vi "Write Image Name.vi"(8 "error in (no error)":errorcluster, 10 "Image Name":string, 11 "CCD in":refnum<class "CCD.lvclass">) -> (0 "error out":errorcluster, 3 "CCD out":refnum<class "CCD.lvclass">)   [LabVIEW 2018, in "CCD.lvclass"]
uses:
  CCD.lvclass
  CCD.lvclass/CCD.ctl
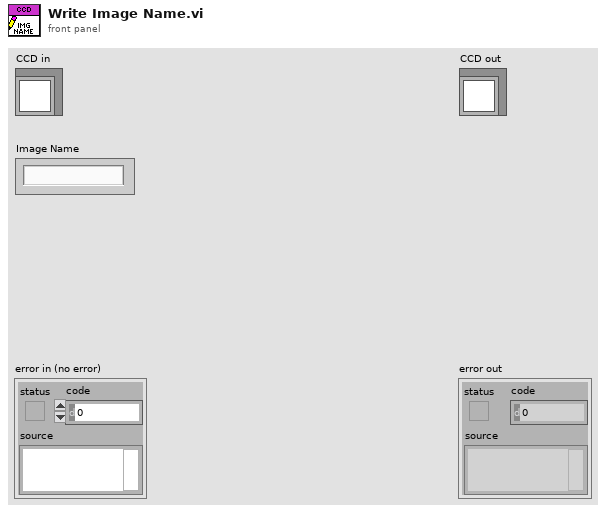
[diagram p1: front panel]
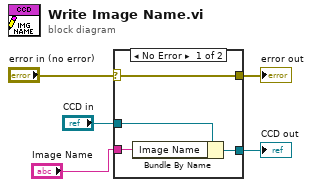
[diagram p0: block diagram]
diagram:
  n1 = case shown="No Error" "error in (no error)" {
    selector: "error in (no error)" -> [w9 w10]
    tunnel: [w9 w10] -> w4
    tunnel: [w7 w11] -> w2
    tunnel: "CCD in" -> [w8 w11]
    tunnel: "Image Name" -> [w6 _]
    frame No Error {
      n2 = Bundle By Name(cluster=w8, "Image Name"=w6) -> (w7:refnum<class "CCD.lvclass">)
    }
    frame Error {
    }
  }
  "error out" <- w4
  "CCD out" <- w2
